vi "Count Leading Zeros.vi"(0 "Array Num":i8[](array[numeric])) -> (1 "Array Dup":i8[](array[numeric]), 2 "NonZero Count":i32)   [LabVIEW 2025]
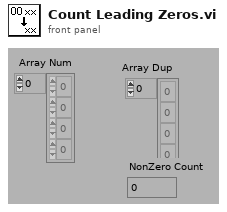
[diagram p1: front panel]
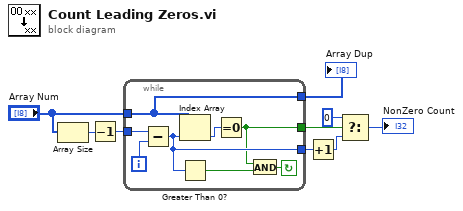
[diagram p0: block diagram]
diagram:
  n1 = Array Size(array="Array Num") -> (size(s)=w8:i32)
  n2 = Decrement(x=w8) -> (x-1=w5:i32)
  n3 = while {
    tunnel: [w10] -> w4
    tunnel: [w11] -> w6
    tunnel: [w12] -> w9
    tunnel: w5 -> [w17]
    tunnel: "Array Num" -> [w11]
    i -> [w13]
    stop <- w16 continue-if-true
    n4 = Subtract(x=w17, y=w13) -> (x-y=w12:i32)
    n5 = Index Array(array=w11, index=w12) -> (element=w15:i8)
    n6 = Greater Than 0?(x=w12) -> (x > 0?=w14:bool)
    n7 = Equal To 0?(x=w15) -> (x = 0?=w10:bool)
    n8 = And(x=w10, y=w14) -> (x .and. y?=w16:bool)
  }
  "Array Dup" <- w6
  n9 = Increment(x=w9) -> (x+1=w3:i32)
  n10 = Select(t=0, s=w4, f=w3) -> (s? t:f=→"NonZero Count":i32)
